vi "Driver jsObject.vi"(8 "error in (no error)":errorcluster, 9 "Station Record (empty)":T1, 10 "Driver jsObject Name (\"\")":string, 11 "Previous String (\"\")":string) -> (0 "error out":errorcluster, 3 "Driver jsObject":string)   [LabVIEW 2011]
uses:
  Driver Record.ctl
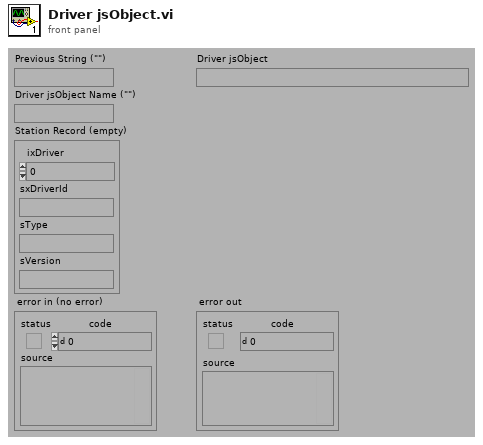
[diagram p1: front panel]
types:
  T1 = typedef "Driver Record.ctl" = cluster{"ixDriver":i32, "sxDriverId":string, "sType":string, "sVersion":string}
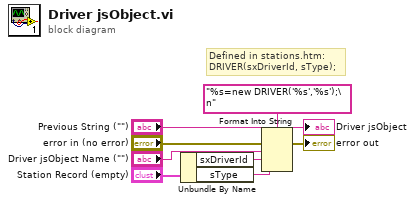
[diagram p0: block diagram]
diagram:
  # "Defined in stations.htm:\nDRIVER(sxDriverId, sType);"
  n1 = Unbundle By Name("Station Record (empty)") -> ("sxDriverId"=w8:string, "sType"=w7:string)
  n2 = Format Into String(format string="%s=new DRIVER('%s','%s');\n", initial string="Previous String (\"\")", error in="error in (no error)", "Driver jsObject Name (\"\")", w8, w7) -> (resulting string=→"Driver jsObject":string, error out=→"error out":errorcluster)
